vi "Linear_regression_with_boston_data.vi"() -> ()   [LabVIEW 2020]
doc: "Using a linear regression on the boston dataset."
uses:
  Model/Supervised/Linear_model/LinearRegressors/LinearRegression/Controls/linear_regression_params.ctl
  Model/Supervised/Linear_model/LinearRegressors/LinearRegression/LinearRegression.lvclass
  C:/Users/cipop/TDF Dropbox/2_Technologies de France/1 - Services et Etudes/PLAIY/2 - DEV/PLAIYLAB/code/Model/Model.lvclass
  Model/Supervised/Linear_model/LinearRegressors/LinearRegression/LinearRegression.vi
panel:
  out "error out":errorcluster caption="sortie d'erreur"
  in  "params":T1={"fit_intercept"=TRUE, "normalize"=FALSE, "copy_X"=TRUE, "n_jobs"=1.0, "positive"=FALSE}
  out "XY Graph":T2(graph)
  out "score":dbl
  out "y":dbl[][](array[numeric])
  out "X":dbl[][](array[numeric])
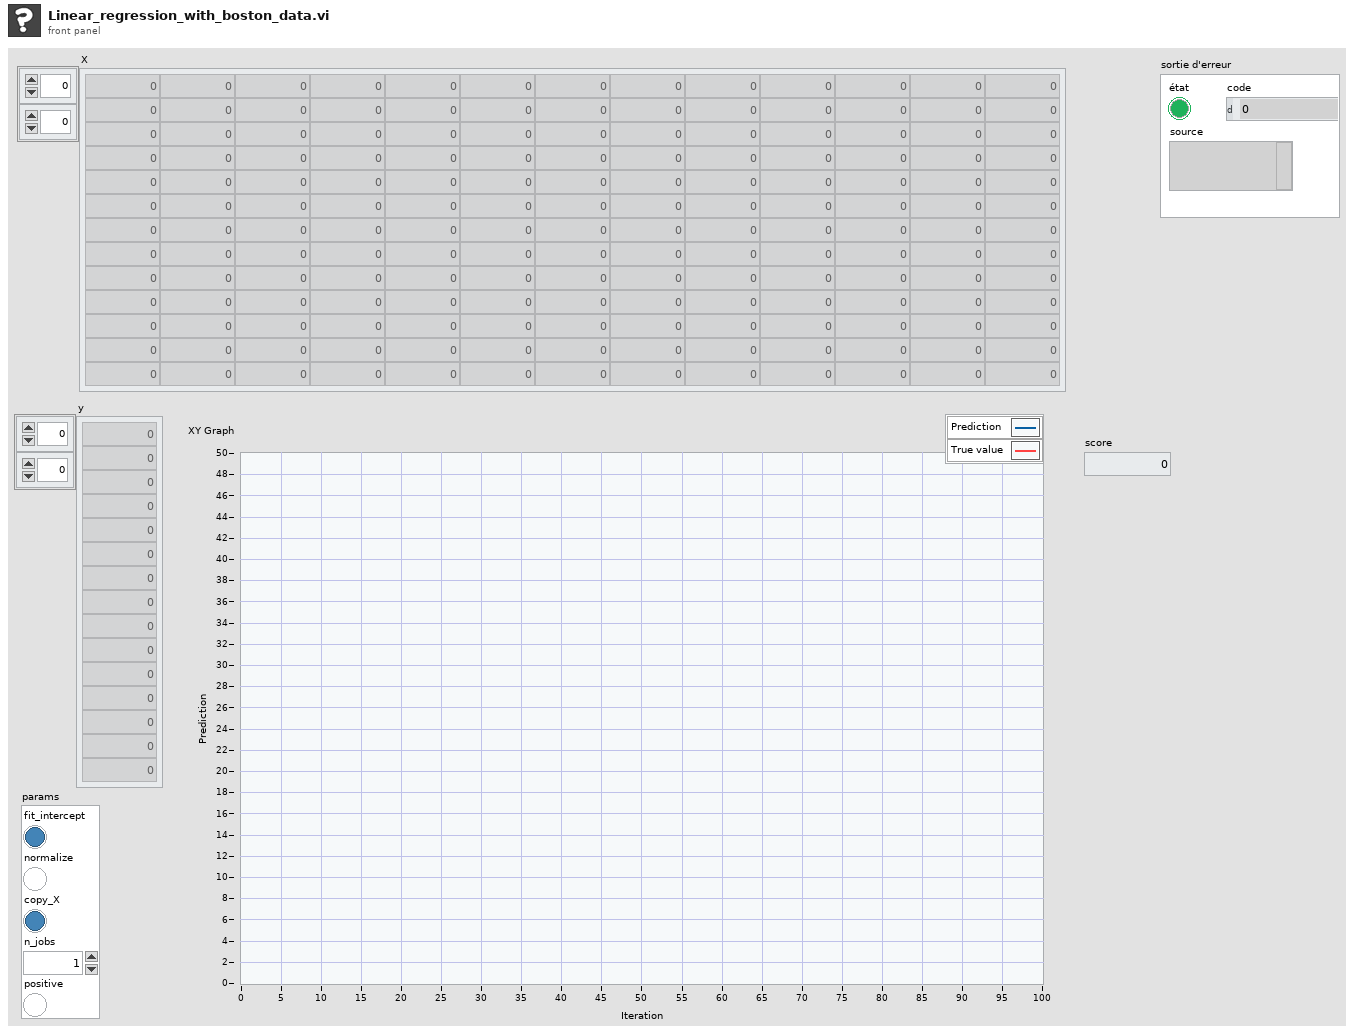
[diagram p1: front panel]
types:
  T1 = typedef "linear_regression_params.ctl" = cluster{"fit_intercept":bool, "normalize":bool, "copy_X":bool, "n_jobs":dbl, "positive":bool}
  T2 = cluster{"XY Graph":cluster{"X":dbl, "Y":dbl}[]}[]
  T3 = cluster{"X Train":dbl[][], "X Test":dbl[][], "Y Train":dbl[][], "Y Test":dbl[][]}
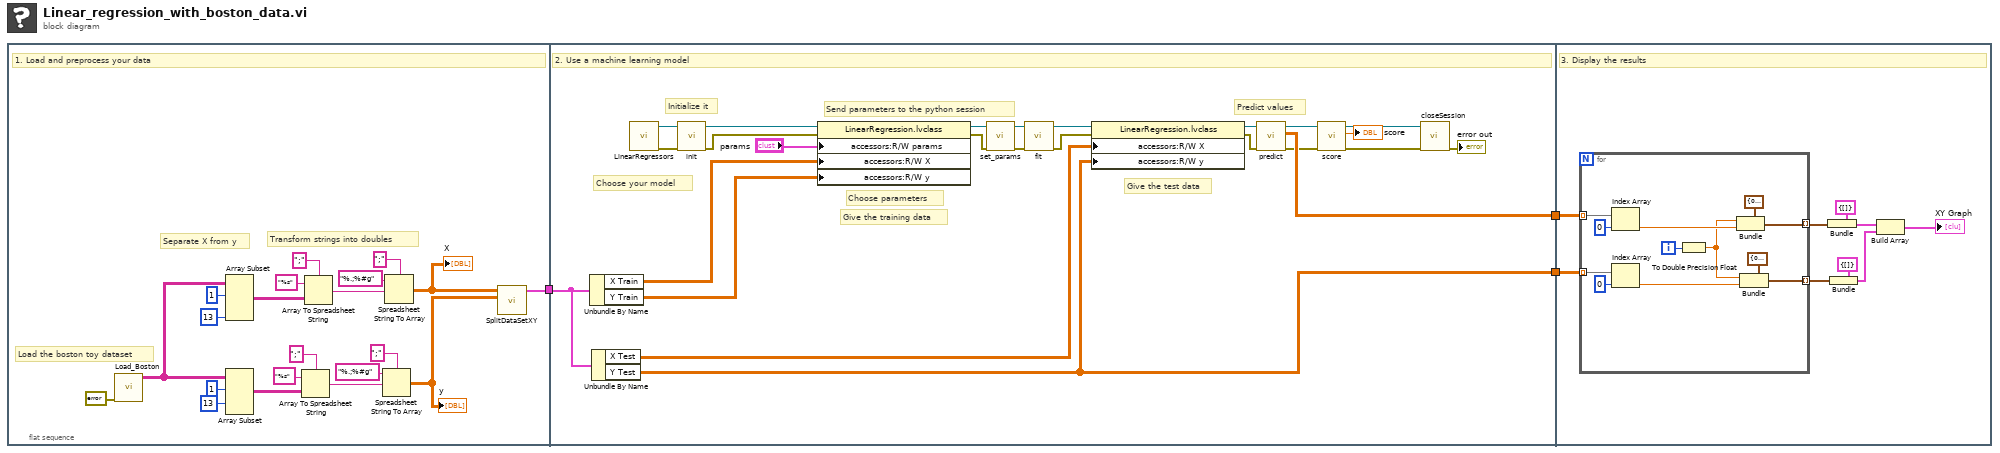
[diagram p0: block diagram]
diagram:
  n1 = flat-sequence {
    tunnel: [w4] -> w2
    tunnel: [w42] -> w3
    tunnel: w2 -> [w40]
    tunnel: [w29] -> w1
    tunnel: w3 -> [w58]
    tunnel: w1 -> [w53]
    frame #0 {
      # "Transform strings into doubles"
      # "Separate X from y"
      # "Load the boston toy dataset"
      # "1. Load and preprocess your data"
      n2 = call "Load_Boston.vi"("error in"=errorcluster {"status"=FALSE, "code"=0, "source"=""}) -> ("Tableau"=w19:string[][])  [unwired: 9 in, 1 out]
      n3 = Array Subset(array=w19, index (row)=1 ("index"), length (col)=13 ("length")) -> (w18:string[][])  [unwired: 2 in]
      n4 = Array Subset(array=w19, index (row)=1 ("index"), index (col)=13 ("index")) -> (w7:string[][])  [unwired: 2 in]
      n5 = Array To Spreadsheet String(delimiter (Tab)=";", array=w7, 3:"%s" ("format string")) -> (spreadsheet string=w8:string)
      n6 = Array To Spreadsheet String(delimiter (Tab)=";", array=w18, 3:"%s" ("format string")) -> (spreadsheet string=w13:string)
      n7 = Spreadsheet String To Array(delimiter (Tab)=";", format string="%.;%#g", spreadsheet string=w8) -> (array=w5:dbl[][])  [unwired: 1 in]
      "y" <- w5
      n8 = Spreadsheet String To Array(delimiter (Tab)=";", format string="%.;%#g", spreadsheet string=w13) -> (array=w6:dbl[][])  [unwired: 1 in]
      "X" <- w6
      n9 = call "SplitDataSetXY.vi"("Y"=w5, "X"=w6) -> ("Split"=w4:T3)  [unwired: 8 in, 1 out]
    }
    frame #1 {
      # "Predict values"
      # "Give the test data"
      # "Send parameters to the python session"
      # "Give the training data"
      # "Choose parameters"
      # "Initialize it"
      # "Choose your model"
      # "2. Use a machine learning model"
      n10 = Unbundle By Name(w40) -> ("X Train"=w41:dbl[][], "Y Train"=w30:dbl[][])
      n11 = Unbundle By Name(w40) -> ("X Test"=w37:dbl[][], "Y Test"=w29:dbl[][])
      n12 = call-poly "LinearRegressors.vi"() -> ("error out"=w25:errorcluster, "out"=w45:refnum<class "LinearRegression.lvclass">)  [unwired: 10 in]
      n13 = call-dynamic "init.vi"("error in (no error)"=w25, "Model en entrée"=w45) -> ("error out"=w49:errorcluster, "Model en sortie"=w48:refnum<class "LinearRegression.lvclass">)  [unwired: 8 in]
      n14 = property class="LinearRegression.lvclass"(reference=w48, error in=w49, "accessors:R/W params"="params", "accessors:R/W X"=w41, "accessors:R/W y"=w30) -> (reference out=w47:refnum<class "LinearRegression.lvclass">, error out=w46:errorcluster)
      n15 = call-dynamic "set_params.vi"("error in (no error)"=w46, "LinearRegression.lvclass 2"=w47) -> ("error out"=w43:errorcluster, "LinearRegression.lvclass"=w44:refnum<class "LinearRegression.lvclass">)  [unwired: 8 in]
      n16 = call-dynamic "fit.vi"("error in (no error)"=w43, "LinearRegression.lvclass 2"=w44) -> ("error out"=w38:errorcluster, "LinearRegression.lvclass"=w39:refnum<class "LinearRegression.lvclass">)  [unwired: 8 in]
      n17 = property class="LinearRegression.lvclass"(reference=w39, error in=w38, "accessors:R/W X"=w37, "accessors:R/W y"=w29) -> (reference out=w35:refnum<class "LinearRegression.lvclass">, error out=w36:errorcluster)
      n18 = call-dynamic "predict.vi"("error in (no error)"=w36, "LinearRegression.lvclass 2"=w35) -> ("error out"=w32:errorcluster, "C"=w42:dbl[][], "LinearRegression.lvclass"=w34:refnum<class "LinearRegression.lvclass">)  [unwired: 7 in]
      n19 = call-dynamic "score.vi"("error in (no error)"=w32, "LinearRegression.lvclass 2"=w34) -> ("error out"=w27:errorcluster, "score"=→"score":dbl, "LinearRegression.lvclass"=w33:refnum<class "LinearRegression.lvclass">)  [unwired: 7 in]
      n20 = call-dynamic "closeSession.vi"("error in"=w27, "Python en entrée"=w33) -> ("error out"=→"error out":errorcluster)  [unwired: 8 in, 1 out]
    }
    frame #2 {
      # "3. Display the results"
      n21 = for {
        tunnel: w58 -> [w70] mode=indexing
        tunnel: w53 -> [w67] mode=indexing
        tunnel: [w60] -> w52 mode=indexing
        tunnel: [w59] -> w51 mode=indexing
        i -> [w64]
        n22 = Index Array(array=w70, index=0) -> (element=w63:dbl)
        n23 = Index Array(array=w67, index=0) -> (element=w61:dbl)
        n24 = To Double Precision Float(number=w64) -> (double precision float=w62:dbl)
        n25 = Bundle(cluster=cluster{"X":dbl, "Y":dbl} {"X"=0.0, "Y"=0.0}, "X"=w62, "Y"=w63) -> (w60:cluster{"X":dbl, "Y":dbl})
        n26 = Bundle(cluster=cluster{"X":dbl, "Y":dbl} {"X"=0.0, "Y"=0.0}, "X"=w62, "Y"=w61) -> (w59:cluster{"X":dbl, "Y":dbl})
      }
      n27 = Bundle(cluster=cluster{"XY Graph":cluster{"X":dbl, "Y":dbl}[]} {"XY Graph"=[]}, "XY Graph"=w52) -> (w55:cluster{"XY Graph":cluster{"X":dbl, "Y":dbl}[]})
      n28 = Bundle(cluster=cluster{"XY Graph":cluster{"X":dbl, "Y":dbl}[]} {"XY Graph"=[]}, "XY Graph"=w51) -> (w54:cluster{"XY Graph":cluster{"X":dbl, "Y":dbl}[]})
      n29 = Build Array(w55, w54) -> (→"XY Graph":T2)
    }
  }
